vi "Change Acquisition Settings.vi"() -> ()   [LabVIEW 2009]
uses:
  Acquisition Settings.vi
panel:
  in  "Tab Control":T1(tab)
  in  "Buffer Size":i32=1000000
  in  "Buffer Mode":u32(ring)=25 items=["yes", "no", "positive", "negative", "high", "low", "low to high", "high to low", "default", "max timebase", "other counter gate", "other counter TC", "other counter output", "other counter source", "source", "gate", "aux line", "in start trigger", "in stop trigger", "automatic", "enabled", "count up", "count down", "hardware", "single", "double", "pulse", "toggle", "quadrature encoder X1", "quadrature encoder X2", "quadrature encoder X4", "two pulse counting", "A high B high", "A high B low", "A low B high", "A low B low", "PFI n", "RTSI n", "timebase n"]
  in  "Arrival Time Settings":T2(array[cluster])=[{"Name"="Ch 1", "Device Number"=2, "Counter Number"=0, "Line Type for Gate"=36, "Line Number for Gate"=30, "Line Type for Source"=9, "Line Number for Source"=0, "Transfer Method"=47, "Signal Routing Configuration"=0}, {"Name"="Ch 2", "Device Number"=2, "Counter Number"=1, "Line Type for Gate"=36, "Line Number for Gate"=34, "Line Type for Source"=9, "Line Number for Source"=0, "Transfer Method"=47, "Signal Routing Configuration"=0}, {"Name"="Ch 3", "Device Number"=1, "Counter Number"=0, "Line Type for Gate"=36, "Line Number for Gate"=30, "Line Type for Source"=37, "Line Number for Source"=7, "Transfer Method"=47, "Signal Routing Configuration"=0}, {"Name"="Ch 4", "Device Number"=1, "Counter Number"=1, "Line Type for Gate"=36, "Line Number for Gate"=34, "Line Type for Source"=37, "Line Number for Source"=7, "Transfer Method"=47, "Signal Routing Configuration"=0}] {"Transfer Method" items=["yes", "no", "positive", "negative", "high", "low", "low to high", "high to low", "default", "max timebase", "other counter gate", "other counter TC", "other counter output", "other counter source", "source", "gate", "aux line", "in start trigger", "in stop trigger", "automatic", "enabled", "count up", "count down", "hardware", "single", "continuous", "pulse", "toggle", "quadrature encoder X1", "quadrature encoder X2", "quadrature encoder X4", "two pulse counting", "A high B high", "A high B low", "A low B high", "A low B low", "PFI n", "RTSI n", "timebase n", "disabled", "PXI backplane clock", "counter n output", "(Reserved) pulse per second", "(Reserved) IRIG-B", "(Reserved) seconds", "(Reserved) nano seconds", "interrupts", "dma", "RTSI clock"]; "Line Type for Source" items=["yes", "no", "positive", "negative", "high", "low", "low to high", "high to low", "default", "max timebase", "other counter gate", "other counter TC", "other counter output", "other counter source", "source", "gate", "aux line", "in start trigger", "in stop trigger", "automatic", "enabled", "count up", "count down", "hardware", "single", "double", "pulse", "toggle", "quadrature encoder X1", "quadrature encoder X2", "quadrature encoder X4", "two pulse counting", "A high B high", "A high B low", "A low B high", "A low B low", "PFI n", "RTSI n", "timebase n"]; "Line Type for Gate" items=["yes", "no", "positive", "negative", "high", "low", "low to high", "high to low", "default", "max timebase", "other counter gate", "other counter TC", "other counter output", "other counter source", "source", "gate", "aux line", "in start trigger", "in stop trigger", "automatic", "enabled", "count up", "count down", "hardware", "single", "double", "pulse", "toggle", "quadrature encoder X1", "quadrature encoder X2", "quadrature encoder X4", "two pulse counting", "A high B high", "A high B low", "A low B high", "A low B low", "PFI n", "RTSI n", "timebase n"]}
  in  "Timer Settings":T3={"Device Number"=2, "Counter Number"=2, "Line Type for Source"=9, "Line Number for Source"=0, "Signal Routing Configuration"=0} {"Line Type for Source" items=["yes", "no", "positive", "negative", "high", "low", "low to high", "high to low", "default", "max timebase", "other counter gate", "other counter TC", "other counter output", "other counter source", "source", "gate", "aux line", "in start trigger", "in stop trigger", "automatic", "enabled", "count up", "count down", "hardware", "single", "double", "pulse", "toggle", "quadrature encoder X1", "quadrature encoder X2", "quadrature encoder X4", "two pulse counting", "A high B high", "A high B low", "A low B high", "A low B low", "PFI n", "RTSI n", "timebase n"]}
  in  "Trigger Settings":T4={"Device Number"=2, "Counter Number"=3, "Signal Routing Configuration"=0}
  in  "Pulse Generation Settings":T5(array[cluster])=[{"Name"="", "Device Number"=2, "Counter Number"=4, "Pulse Spec 1 (Clocks)"=40, "Pulse Spec 2 (Clocks)"=40, "Signal Routing Configuration"=0, "Inverted"=FALSE}]
  in  "AO Definitions":T6(array[cluster]) {"clock source (internal:1)" items=["no change", "internal", "counter 1", "counter 2", "counter 3", "counter 5", "I/O connector", "RTSI connection", "PFI pin, low to high", "PFI pin, high to low", "RTSI pin, low to high", "RTSI pin, high to low", "GPCTR 1 output, low to high", "GPCTR 1 output, high to low", "ATCOUT, low to high", "ACTOUT, high to low", "internal clock 2"]; "Signal Description"."period" format="%.2f"; "Signal Description"."% duty cycle" format="%.2f"; "Signal Description"."resting voltage" format="%.2f"; "Signal Description"."phase (0 deg)" format="%.2f"; "Signal Description"."offset (0.0)" format="%.2f"; "Signal Description"."amplitude" format="%.2f"}
  in  "Signal Routing Configuration":T7(array[cluster]) {"Signal Routing"."signal source" items=["no change", "none", "AI start trigger", "AI stop trigger", "AI convert", "GPCTR 1 source", "GPCTR 1 gate", "AO update", "AO start trigger", "AI scan start", "GPCTR  0 source", "GPCTR  0 gate", "GPCTR  0 output", "RTSI 0", "RTSI 1", "RTSI 2", "RTSI 3", "RTSI 4", "RTSI 5", "RTSI 6", "RTSI clock", "board clock", "PLL input pin", "marker out", "SYNC out", "analog trigger circuit output", "end of acquisition", "frequency output", "high", "low", "SCANCLK", "inverted voltmeter complete", "voltmeter complete", "GPCTR n source", "GPCTR n gate", "GPCTR n output", "PFI n", "AI scan in progress", "(Reserved_1)", "(Reserved_2)", "stable 10MHz", "PXI Star"]; "Signal Routing"."signal name" items=["no change", "PFI 0", "PFI 1", "PFI 2", "PFI 3", "PFI 4", "PFI 5", "PFI 6", "PFI 7", "PFI 8", "PFI 9", "GPCTR 0 output", "RTSI 0", "RTSI 1", "RTSI 2", "RTSI 3", "RTSI 4", "RTSI 5", "RTSI 6", "RTSI clock", "board clock", "PLL reference clock", "SCANCLK", "I/O connector", "PFI n", "start trigger", "configurable filter", "PXI backplane clock", "PXI Star n"]}
  in  "Cancel":bool
  in  "OK":bool
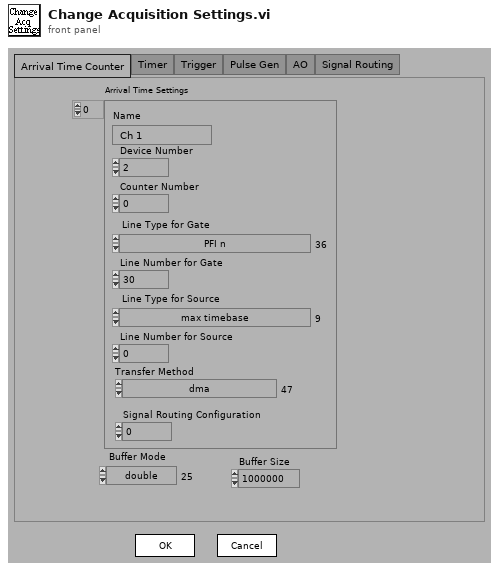
[diagram p1: front panel]
types:
  T1 = enum32{"Arrival Time Counter", "Timer", "Trigger", "Pulse Gen", "AO", "Signal Routing"}
  T2 = cluster{"Name":string, "Device Number":i16, "Counter Number":i16, "Line Type for Gate":u32, "Line Number for Gate":u32, "Line Type for Source":u32, "Line Number for Source":u32, "Transfer Method":u32, "Signal Routing Configuration":i16}[]
  T3 = cluster{"Device Number":i16, "Counter Number":i16, "Line Type for Source":u32, "Line Number for Source":u32, "Signal Routing Configuration":i16}
  T4 = cluster{"Device Number":i16, "Counter Number":i16, "Signal Routing Configuration":i16}
  T5 = cluster{"Name":string, "Device Number":i16, "Counter Number":i16, "Pulse Spec 1 (Clocks)":u32, "Pulse Spec 2 (Clocks)":u32, "Signal Routing Configuration":i16, "Inverted":bool}[]
  T6 = cluster{"device":i16, "channel":tag, "buffer size":i32, "Signal Description":cluster{"Name":string, "signal type":enum16{"Sine Wave", "Square Wave", "Sawtooth", "Triangle Wave"}, "period":dbl, "amplitude":dbl, "phase (0 deg)":dbl, "offset (0.0)":dbl, "resting voltage":dbl, "% duty cycle":dbl}[], "clock source (internal:1)":u16, "Clock Line Number":i16}[]
  T7 = cluster{"Name":string, "Signal Routing":cluster{"signal name":u16, "signal source":u16, "signal source line number":u32, "signal name line number":u32}[]}[]
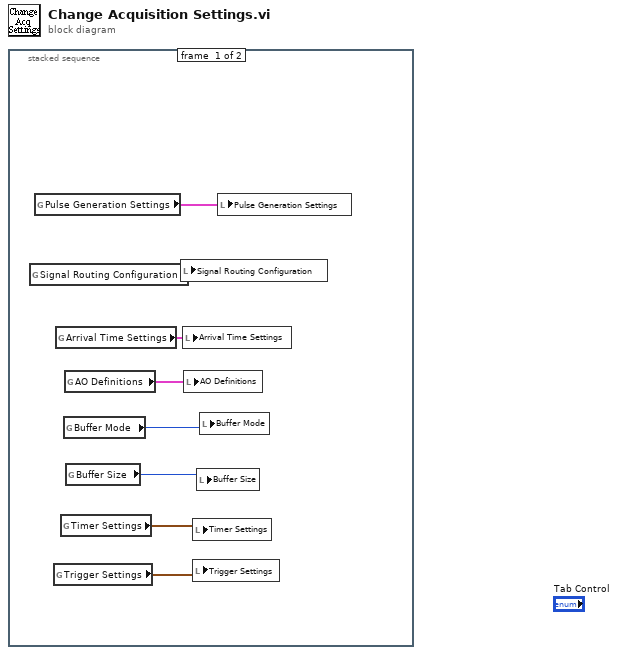
[diagram p0: block diagram]
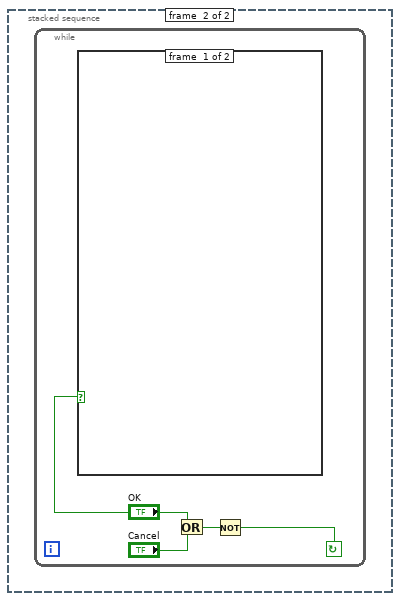
[diagram p2: hidden frame]
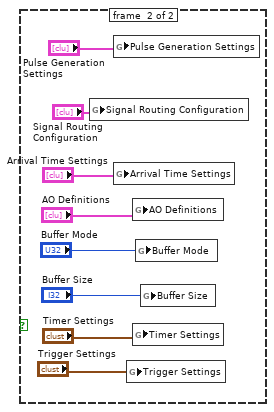
[diagram p3: hidden frame]
diagram:
  n1 = stacked-sequence {
    frame #0 {
      n2 = global read "Acquisition Settings.vi" "Signal Routing Configuration"() -> (w1:T7)
      n3 = global read "Acquisition Settings.vi" "Pulse Generation Settings"() -> (w2:T5)
      n4 = global read "Acquisition Settings.vi" "Trigger Settings"() -> (w4:T4)
      n5 = global read "Acquisition Settings.vi" "Arrival Time Settings"() -> (w8:T2)
      n6 = global read "Acquisition Settings.vi" "Timer Settings"() -> (w5:T3)
      n7 = global read "Acquisition Settings.vi" "Buffer Mode"() -> (w7:u32)
      n8 = global read "Acquisition Settings.vi" "AO Definitions"() -> (w3:T6)
      n9 = global read "Acquisition Settings.vi" "Buffer Size"() -> (w6:i32)
      n10 = local write "Signal Routing Configuration"(w1) -> ()
      n11 = local write "Arrival Time Settings"(w8) -> ()
      n12 = local write "AO Definitions"(w3) -> ()
      n13 = local write "Timer Settings"(w5) -> ()
      n14 = local write "Trigger Settings"(w4) -> ()
      n15 = local write "Buffer Size"(w6) -> ()
      n16 = local write "Buffer Mode"(w7) -> ()
      n17 = local write "Pulse Generation Settings"(w2) -> ()
    }
    frame #1 {
      n18 = while {
        stop <- w9 continue-if-true
        n19 = case shown="True" "OK" {
          frame #0 {
          }
          frame #1 {
            n20 = global write "Acquisition Settings.vi" "Signal Routing Configuration"("Signal Routing Configuration") -> ()
            n21 = global write "Acquisition Settings.vi" "Pulse Generation Settings"("Pulse Generation Settings") -> ()
            n22 = global write "Acquisition Settings.vi" "Arrival Time Settings"("Arrival Time Settings") -> ()
            n23 = global write "Acquisition Settings.vi" "Trigger Settings"("Trigger Settings") -> ()
            n24 = global write "Acquisition Settings.vi" "AO Definitions"("AO Definitions") -> ()
            n25 = global write "Acquisition Settings.vi" "Timer Settings"("Timer Settings") -> ()
            n26 = global write "Acquisition Settings.vi" "Buffer Mode"("Buffer Mode") -> ()
            n27 = global write "Acquisition Settings.vi" "Buffer Size"("Buffer Size") -> ()
          }
        }
        n28 = Or(x="OK", y="Cancel") -> (x .or. y?=w10:bool)
        n29 = Not(x=w10) -> (.not. x?=w9:bool)
      }
    }
  }
